vi "test String to I32_2.vi"(11 "Test Case In":refnum<class "test Electronic Datasheet.lvclass">) -> (0 "error out":errorcluster, 3 "Test Case Out":refnum<class "test Electronic Datasheet.lvclass">)   [LabVIEW 2024, in "Test Utilities.lvclass"]
uses:
  Test Utilities.lvclass
  Test Utilities.lvclass/Test Utilities.ctl
  10210a59-fd71-4d7c-8873-a3b2364ddadf.vi
  source/CANopen.lvlib
  EDS-File-Viewer/Tests/source/test Electronic Datasheet/test Electronic Datasheet.lvclass
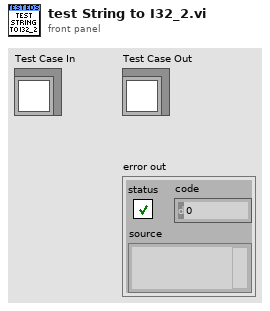
[diagram p1: front panel]
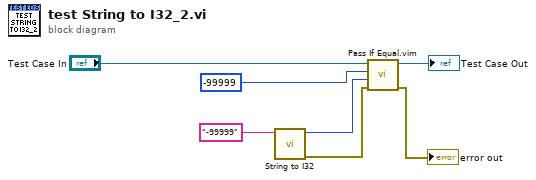
[diagram p0: block diagram]
diagram:
  n1 = call "String to I32.vi"("Integer String"="-99999" ("String")) -> ("error out"=w3:errorcluster, "I32"=w2:i32)  [unwired: 9 in]
  n2 = call "Pass If Equal.vim"("error in (no error)"=w3, "Actual"=w2, "Expected"=-99999, "LUnit Test Case In"="Test Case In") -> ("error out"=→"error out":errorcluster, "LUnit Test Case Out"=→"Test Case Out":refnum<class "test Electronic Datasheet.lvclass">)  [unwired: 6 in]
